vi "Open.vi"(5 "Global Timeout [mSec] (-1)":i32, 6 "VI":refnum<vi>, 7 "Delay mSec (0)":u32, 8 "error in (no error)":errorcluster, 9 "Explorer Visible? (F)":bool, 10 "Window Title":string="Action Status", 11 "Bar in":refnum<class "Bar.lvclass">) -> (0 "error out":errorcluster, 3 "Bar out":refnum<class "Bar.lvclass">)   [LabVIEW 2015, in "Simple Progress Bar.lvlib" / "Bar.lvclass"]
doc: "Open the progress bar user interface.\n\n<b>Global Timeout</b> duration in mSec will automatically close the window if the process has not finished before."
uses:
  Bar.lvclass
  Bar.lvclass/Bar.ctl
  Simple Progress Bar.lvlib
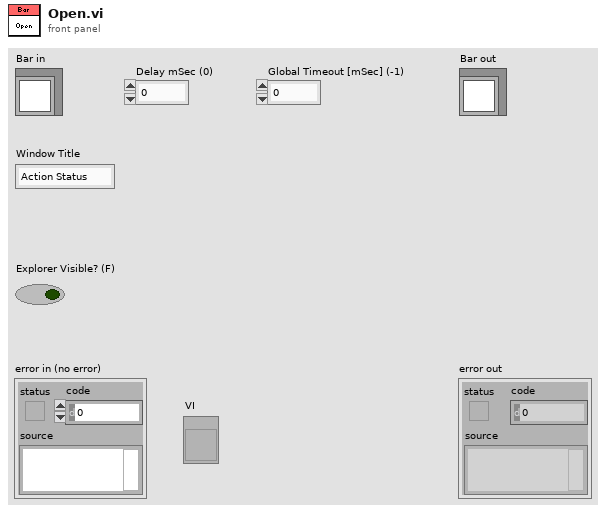
[diagram p1: front panel]
types:
  T1 = enum32{"Invalid", "Standard", "Closed", "Hidden", "Minimized", "Maximized"}
  T2 = typedef "Simple Progress Bar.lvlib/UI Events.ctl" = cluster{"Done":refnum<user-event>, "Cancel":refnum<user-event>, "Explore":refnum<user-event>}
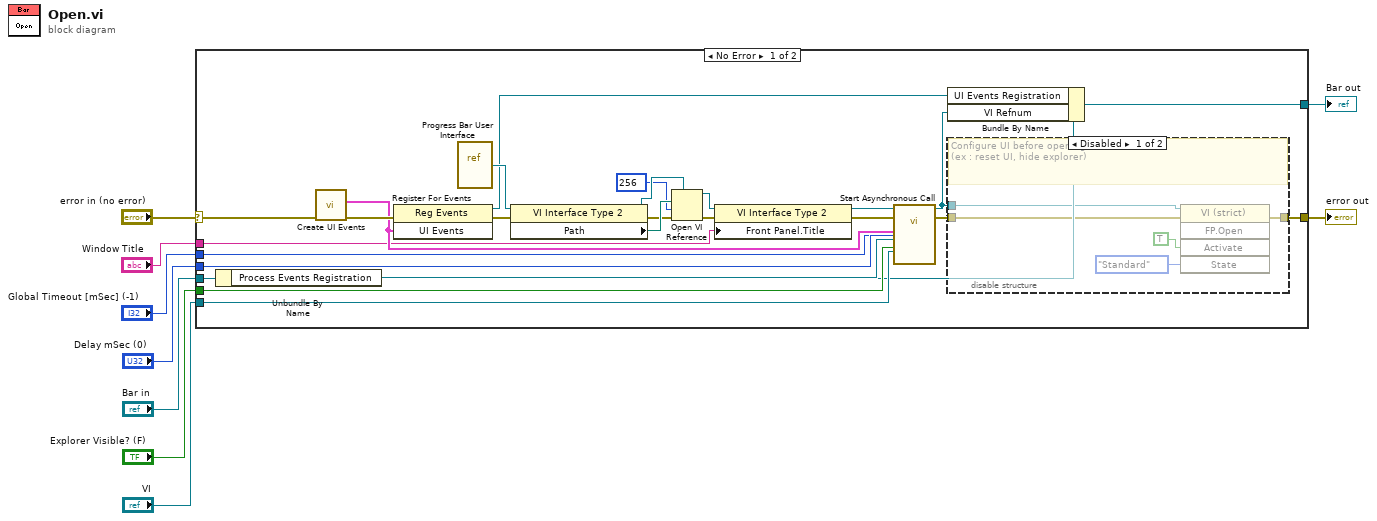
[diagram p0: block diagram]
diagram:
  n1 = case shown="No Error" "error in (no error)" {
    selector: "error in (no error)" -> [w24 w42]
    tunnel: [w28 w42] -> w7
    tunnel: "Explorer Visible? (F)" -> [w23 _]
    tunnel: "Window Title" -> [w18 _]
    tunnel: "VI" -> [w17 _]
    tunnel: "Delay mSec (0)" -> [w16 _]
    tunnel: "Bar in" -> [w14 w41]
    tunnel: [w13 w41] -> w2
    tunnel: "Global Timeout [mSec] (-1)" -> [w10 _]
    frame No Error {
      n2 = Unbundle By Name(w14) -> ("Process Events Registration"=w15:refnum<event-registration>)
      n3 = call "Create UI Events.vi"("error in (no error)"=w24) -> ("error out"=w27:errorcluster, "UI Events"=w25:T2)  [unwired: 9 in]
      n4 = register-events(error in=w27, w25) -> (reference out=w12:refnum<event-registration>, error out=w26:errorcluster)  [unwired: 1 in]
      n5 = vi-ref "Progress Bar User Interface.vi"() -> (w34:refnum<vi>)
      n6 = property class="VI Interface Type 2"(reference=w34, error in=w26) -> (reference out=w31:refnum<vi>, error out=w32:errorcluster, "Path"=w33:path)
      n7 = Open VI Reference(type specifier VI Refnum (for type only)=w31, vi path=w33, options=256, error in (no error)=w32) -> (vi reference=w20:refnum<vi>, error out=w30:errorcluster)  [unwired: 2 in]
      n8 = property class="VI Interface Type 2"(reference=w20, error in=w30, "Front Panel.Title"=w18) -> (reference out=w19:refnum<vi>, error out=w21:errorcluster)
      n9 = call-by-ref "Start Asynchronous Call"(reference=w19, error in=w21, "Global Timeout [mSec] (-1)"=w10, "VI"=w17, "Delay mSec (0)"=w16, "Explorer Visible? (F)"=w23, "Process Events Registration"=w15, "UI Events"=w25) -> (reference out=w11:refnum<vi>, error out=w29:errorcluster)  [unwired: 4 in, 2 out]
      n10 = Bundle By Name(cluster=w14, "UI Events Registration"=w12, "VI Refnum"=w11) -> (w13:refnum<class "Bar.lvclass">)
      n11 = disable-structure shown="Disabled" {
        disable-tunnel: w29 -> [w39 w40]
        disable-tunnel: [w38 w40] -> w28
        disable-tunnel: w11 -> [w37 _]
        frame Disabled {
          # "Configure UI before opening.\n(ex : reset UI, hide explorer)"
          n12 = invoke class="VI (strict)" method="FP.Open"(reference=w37, error in=w39, "Activate"=TRUE ("Activate?"), "State"=T1."Standard") -> (error out=w38:errorcluster)  [unwired: 1 in, 4 out]
        }
        frame Enabled {
        }
      }
    }
    frame Error {
    }
  }
  "error out" <- w7
  "Bar out" <- w2
